vi "HRP Stopwatch.vi"() -> ()   [LabVIEW 2015]
panel:
  out "Seconds":i32
  out "Minutes":i32
  in  "Quit":bool
  in  "Stop":bool
  in  "Start":bool
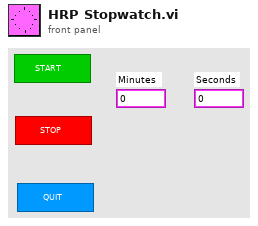
[diagram p1: front panel]
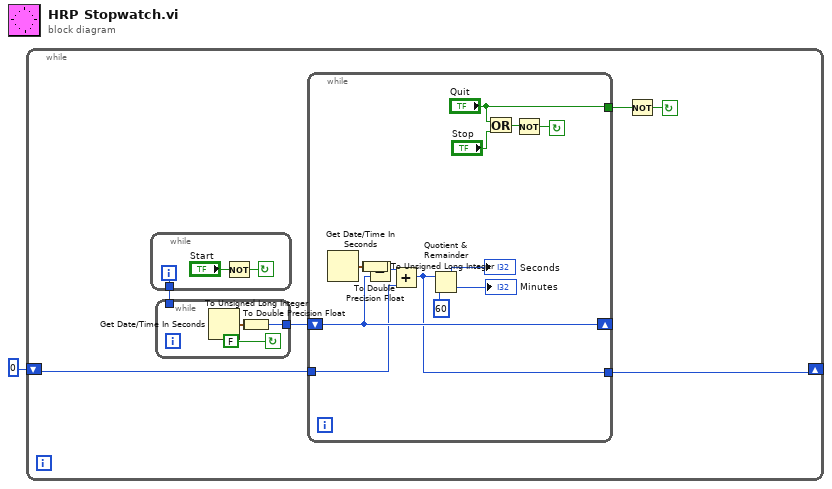
[diagram p0: block diagram]
diagram:
  n1 = while {
    shift-left: 0 -> [w2]
    shift-right: [w3] -> _
    stop <- w4 continue-if-true
    n2 = while {
      tunnel: [w26] -> w6
      i -> [w26]
      stop <- w27 continue-if-true
      n3 = Not(x="Start") -> (.not. x?=w27:bool)
    }
    n4 = while {
      tunnel: [w11] -> w7
      tunnel: w6 -> [_]
      stop <- FALSE continue-if-true
      n5 = Get Date/Time In Seconds() -> (seconds since 1Jan1904=w8:timestamp)
      n6 = To Double Precision Float(number=w8) -> (double precision float=w10:dbl)
      n7 = To Unsigned Long Integer(number=w10) -> (unsigned 32bit integer=w11:u32)
    }
    n8 = while {
      tunnel: w2 -> [w16]
      tunnel: [w14] -> w3
      tunnel: ["Quit"] -> w5
      shift-left: w7 -> [w24]
      shift-right: [w24] -> _
      stop <- w17 continue-if-true
      n9 = Get Date/Time In Seconds() -> (seconds since 1Jan1904=w12:timestamp)
      n10 = To Double Precision Float(number=w12) -> (double precision float=w13:dbl)
      n11 = To Unsigned Long Integer(number=w13) -> (unsigned 32bit integer=w25:u32)
      n12 = Subtract(x=w25, y=w24) -> (x-y=w15:u32)
      n13 = Add(x=w15, y=w16) -> (x+y=w14:u32)
      n14 = Quotient & Remainder(x=w14, y=60) -> (x-y*floor(x/y)=→"Seconds":u32, floor(x/y)=→"Minutes":u32)
      n15 = Or(x="Quit", y="Stop") -> (x .or. y?=w18:bool)
      n16 = Not(x=w18) -> (.not. x?=w17:bool)
    }
    n17 = Not(x=w5) -> (.not. x?=w4:bool)
  }
